vi "Configure Event Search (Serial Bus - IIC).vi"(5 "Data 2 Value (-1)":i32=-1, 6 "Data Value (-1)":i32=-1, 7 "Address (-1)":i32=-1, 8 "error in (no error)":errorcluster, 9 "Qualifier (0: Equal)":i32(ring) items=["Equal", "Not Equal", "Less Than", "Greater Than"], 10 "Search Operation (0: Read 7)":i32(ring) items=["Read 7", "Write 7", "No ACK", "Address No ACK", "Read 7 Data 2", "Write 7 Data 2", "Restart", "Read EEPROM", "Address"], 11 "VISA resource name":refnum<visa-resource-name>) -> (0 "error out":errorcluster, 3 "VISA resource name out":refnum<visa-resource-name>)   [LabVIEW 2015, in "Agilent 2000 3000 X-Series.lvlib"]
doc: "Configures the event search of IIC bus.\n\nNotes:\nThis VI is not supported by EDUX1052A/G, DSOX1202A/G, DSOX1204A/G models."
uses:
  Agilent 2000 3000 X-Series.lvlib
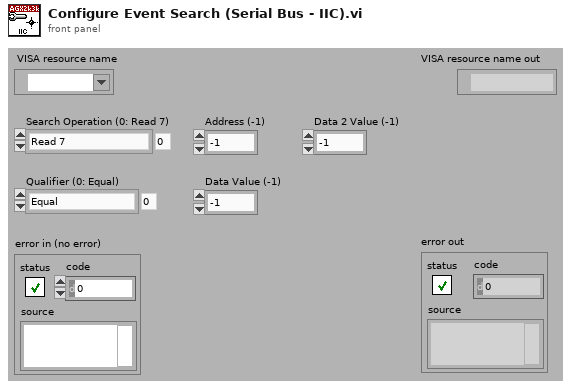
[diagram p1: front panel]
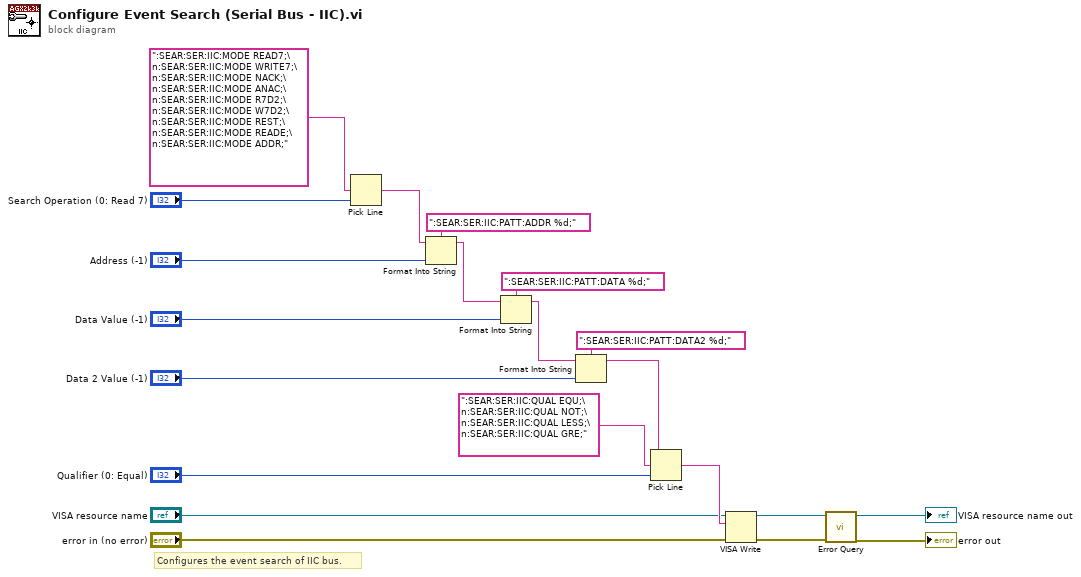
[diagram p0: block diagram]
diagram:
  # "Configures the event search of IIC bus."
  n1 = Pick Line(multi-line string=":SEAR:SER:IIC:MODE READ7;\n:SEAR:SER:IIC:MODE WRITE7;\n:SEAR:SER:IIC:MODE NACK;\n:SEAR:SER:IIC:MODE ANAC;\n:SEAR:SER:IIC:MODE R7D2;\n:SEAR:SER:IIC:MODE W7D2;\n:SEAR:SER:IIC:MODE REST;\n:SEAR:SER:IIC:MODE READE;\n:SEAR:SER:IIC:MODE ADDR;", line index="Search Operation (0: Read 7)") -> (output string=w19:string)  [unwired: 1 out]
  n2 = Format Into String(format string=":SEAR:SER:IIC:PATT:ADDR %d;", initial string=w19, "Address (-1)") -> (resulting string=w16:string)  [unwired: 1 in, 1 out]
  n3 = Format Into String(format string=":SEAR:SER:IIC:PATT:DATA %d;", initial string=w16, "Data Value (-1)") -> (resulting string=w13:string)  [unwired: 1 in, 1 out]
  n4 = Format Into String(format string=":SEAR:SER:IIC:PATT:DATA2 %d;", initial string=w13, "Data 2 Value (-1)") -> (resulting string=w8:string)  [unwired: 1 in, 1 out]
  n5 = Pick Line(string ("")=w8, multi-line string=":SEAR:SER:IIC:QUAL EQU;\n:SEAR:SER:IIC:QUAL NOT;\n:SEAR:SER:IIC:QUAL LESS;\n:SEAR:SER:IIC:QUAL GRE;", line index="Qualifier (0: Equal)") -> (output string=w7:string)
  n6 = VISA Write(VISA resource name="VISA resource name", write buffer=w7, error in (no error)="error in (no error)") -> (VISA resource name out=w4:refnum<visa-resource-name>, error out=w3:errorcluster)  [unwired: 1 out]
  n7 = call "Error Query.vi"("error in (no error)"=w3, "VISA resource name"=w4) -> ("error out"=→"error out":errorcluster, "VISA resource name out"=→"VISA resource name out":refnum<visa-resource-name>)  [unwired: 8 out]
